vi "Tag Convert.vi"(0 "Tree Reference In":refnum<vi>, 2 "InputTag (Current)":string, 5 "error in (no error)":errorcluster, 9 "Column # (0)":i32) -> (14 "Tree Reference Out":refnum<vi>, 16 "Duplicate Tag":string, 17 "Tag Text":string, 19 "error out":errorcluster)   [LabVIEW 2023, in "DSLV_Tree.lvlib"]
doc: "Retrieves the text in column 0 assosciated with the Input Tag or if there is no input, the currently selected item. Ignores the call if no item is selected. Returns error code 1136 if an improper tag is input."
uses:
  DSLV_Tree.lvlib
panel:
  # "VI INPUTS"
  # "VI OUTPUTS"
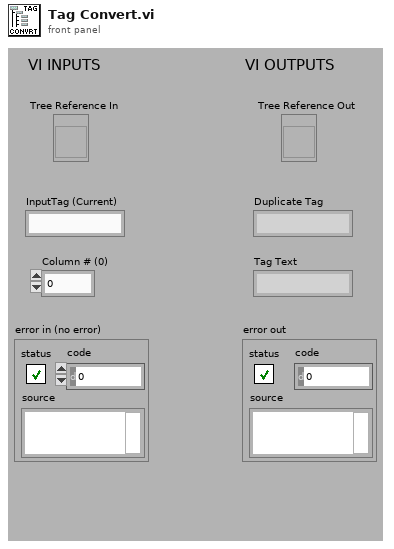
[diagram p1: front panel]
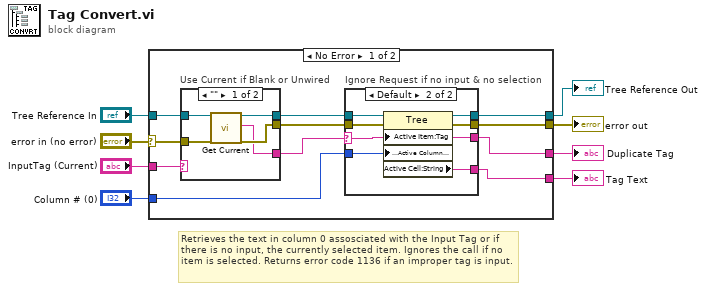
[diagram p0: block diagram]
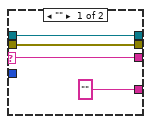
[diagram p3: hidden frame]
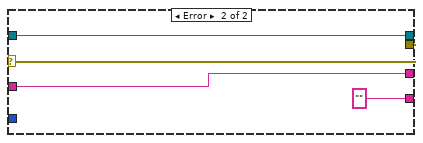
[diagram p4: hidden frame]
diagram:
  # "Retrieves the text in column 0 assosciated with the Input Tag or if there is no input, the currently selected item. Ignores the call if no item is selected. Returns error code 1136 if an improper tag is input."
  n1 = case shown="No Error" "error in (no error)" {
    tunnel: "Tree Reference In" -> [w15 w42]
    selector: "error in (no error)" -> [w13 w41]
    tunnel: [w17 w42] -> w8
    tunnel: [w19 "" ("Cell String")] -> w4
    tunnel: [w18 w41] -> w7
    tunnel: [w16 w40] -> w5
    tunnel: "InputTag (Current)" -> [w14 w40]
    tunnel: "Column # (0)" -> [w9 _]
    frame No Error {
      n2 = case "Use Current if Blank or Unwired" shown="\"\"" w14 {
        selector: w14 -> [_ w25]
        tunnel: [w23 w27] -> w12
        tunnel: w15 -> [w24 w27]
        tunnel: [w22 w26] -> w11
        tunnel: w13 -> [w21 w26]
        tunnel: [w20 w25] -> w10
        frame "" {
          n3 = call "Get Current.vi"("Tree Reference In"=w24, "error in (no error)"=w21) -> ("Tree Reference Out"=w23:refnum<vi>, "Current Tag"=w20:string, "error out"=w22:errorcluster)  [unwired: 14 in, 1 out]
        }
        frame Default {
        }
      }
      n4 = case "Ignore Request if no input & no selection" shown="Default" w10 {
        selector: w10 -> [w29 w33]
        tunnel: w12 -> [w30 w38]
        tunnel: w11 -> [w31 w37]
        tunnel: ["" ("Cell String") w36] -> w19
        tunnel: [w31 w35] -> w18
        tunnel: [w30 w34] -> w17
        tunnel: [w29 w33] -> w16
        tunnel: w9 -> [_ w32]
        frame "" {
        }
        frame Default {
          n5 = property class="Tree"(reference=w38, error in=w37, "Active Item:Tag"=w33, "Active Cell:Active Column Number"=w32) -> (reference out=w34:refnum<vi>, error out=w35:errorcluster, "Active Cell:String"=w36:string)
        }
      }
    }
    frame Error {
    }
  }
  "Tree Reference Out" <- w8
  "error out" <- w7
  "Duplicate Tag" <- w5
  "Tag Text" <- w4
